vi "Arm One Channel.vi"(3 "error IN":errorcluster, 5 "task ID IN":u32 format="%.0x") -> (0 "error out":errorcluster, 2 "task ID out":u32 caption="task ID OUT" format="%.0x")   [LabVIEW 2012]
doc: "DESCRIPTION:\nThis VI arms two counters, using an NI-TIO based device (e.g.: 6602). The counters increments its event count everytime a pulse comes into its source input. The counters only increments between the rising edge of the aux line and the rising edge of the gate. The value of the counter can be read when the counter is finished or an error occurs. \n\n\n\nINSTRUCTIONS:\n1. Enter the device and counter you want use.\n\n3. Connect your signals as described below in I/O CONNECTIONS.\n4. Run the VI.\n\n\nKEY PARAMETERS:\nCounter Group Config.vi: task type = two edge separation measurement\nCounter Source (NI-TIO).vi: Source Specification\nCounter Gate (NI-TIO).vi: Gate Specification\nCounter Aux Line (NI-TIO): Aux Line Specification\nCounter Get Attribute.vi: armed, TC Reached, count\nCounter Control.vi: Program, Reset\n\n\n\nI/O CONNECTIONS:\nConnect the start signal to the aux line input of the selected counter. Connect the stop signal to the gate input of the selected counter. \nIf you selected the Source Selection to be \"PFI line\", connect your event count base signal to the PFI line indicated by \"Source PFI line number used\". (If you selected \"Internal Timebase\", no source connection is necessary.)\n\nNOTE: For actual I/O pin numbers, please refer to your hardware user manual.\n\n\n\nDAQ VIs USED:\nCounter Group Config.vi\nCounter Source (NI-TIO).vi\nCounter Gate (NI-TIO).vi\nCounter Aux Line (NI-TIO)\nCounter Get Attribute.vi\nCounter Control.vi"
panel:
  # "For instructions select\nFile >> VI Properties >> Documentation"
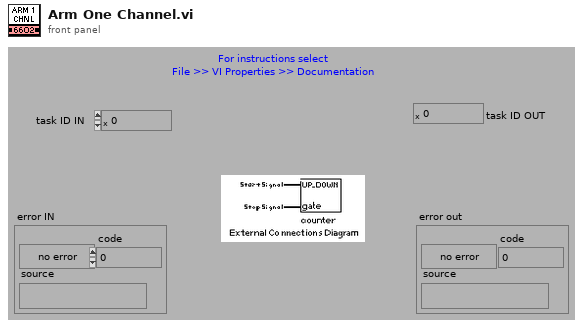
[diagram p1: front panel]
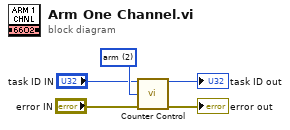
[diagram p0: block diagram]
diagram:
  w5 = u32 2 items=["program", "reset", "arm", "prepare", "disarm", "count up", "count down", "switch cycle", "snapshot"] ("control code")
  n1 = call "Counter Control.vi"("task ID"="task ID IN", "control code"=w5, "error in (no error)"="error IN") -> ("task ID out"=→"task ID out":u32, "error out"=→"error out":errorcluster)  [unwired: 11 in]
